vi "Add_to_speed_calib_file.vi"(2 "Desired Velocity":dbl format="%.2f", 3 "Max Velocity":dbl format="%.2f", 4 "New Row":dbl[](array[numeric]) format="%.2f", 5 "Max % Tweak allowable":dbl=40.0, 6 "Rig Name":string, 7 "Mode":enum16{"Add Row", "Get Error Value"}(ring)) -> (0 "Tweaked Demand":dbl format="%.4f", 1 "Calib Tweak %":dbl format="%.4f")   [LabVIEW 2022 SP3]
uses:
  Anemometry/Anemometry Sub Vis/File/Setup_Filetype.ctl
  Anemometry/Anemometry Sub Vis/Controls/In_Range.ctl
panel:
  out "XY Graph":T1(graph)
  out "Array":dbl[][](array[numeric]) format="%.4f"
  out "Channel Values":string[][](array[string])
  # "Dem Vel       Calib Tweak   Meas Vel"
  # "Dem V        Tweak      Weighting"
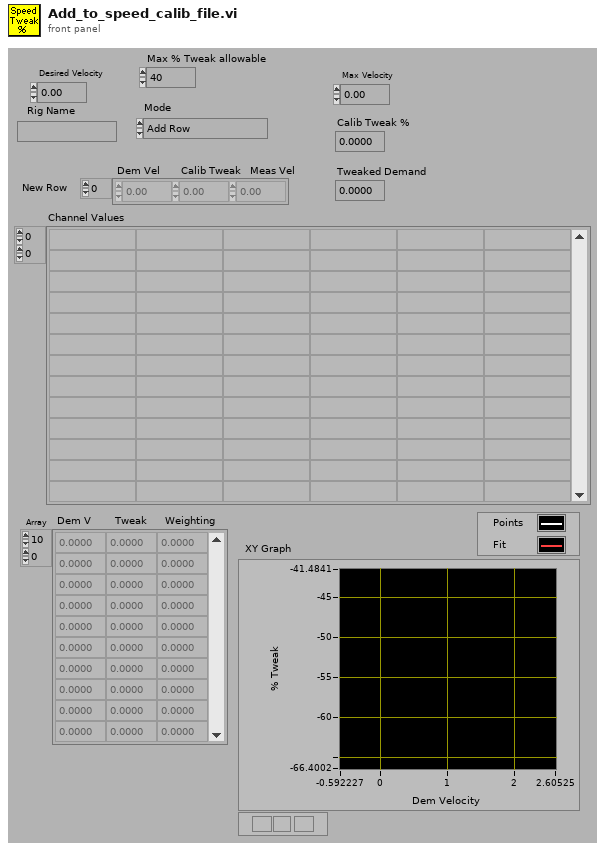
[diagram p1: front panel]
types:
  T1 = cluster{"t":dbl[], "Best Polynomial Fit":dbl[]}[]
  T2 = typedef "Setup_Filetype.ctl" = enum16{"Measurement Setups", "Calibration Setups", "General", "Results File Plotter Setups", "Speed Calib Tweaks"}
  T3 = typedef "In_Range.ctl" = enum16{"%", "±", "% & ±"}
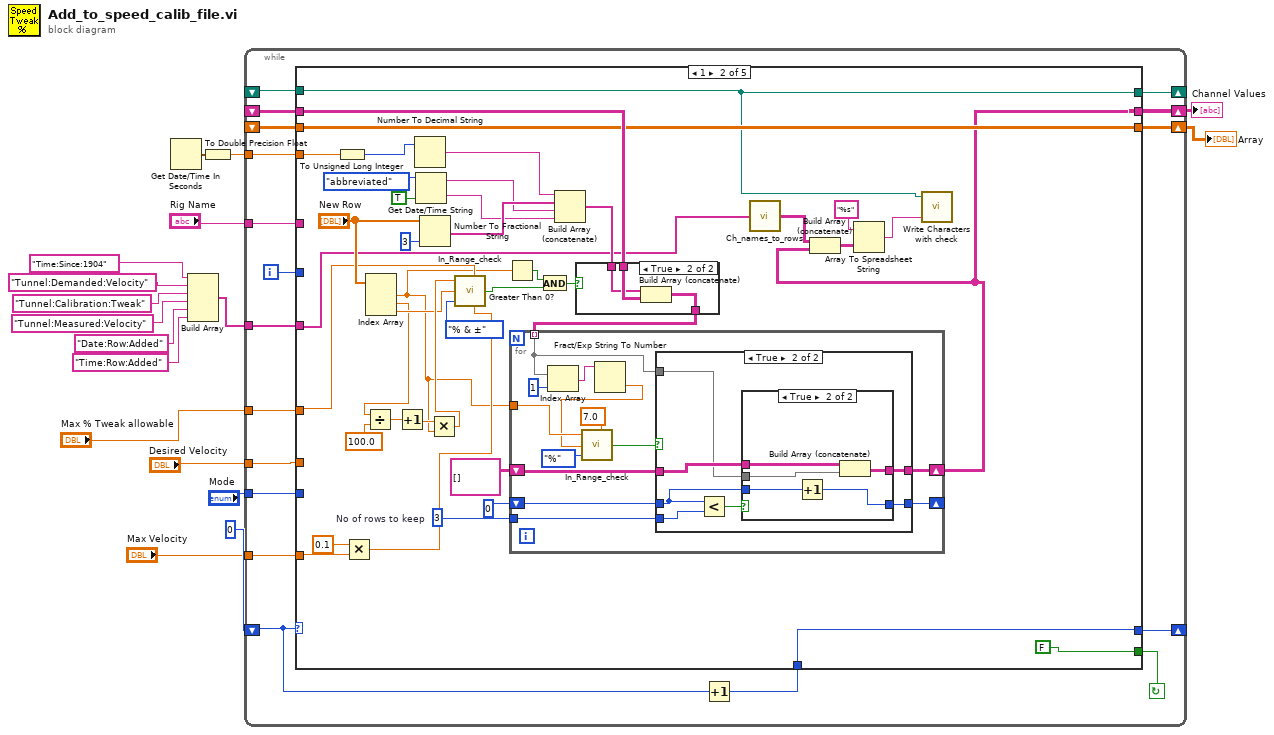
[diagram p0: block diagram]
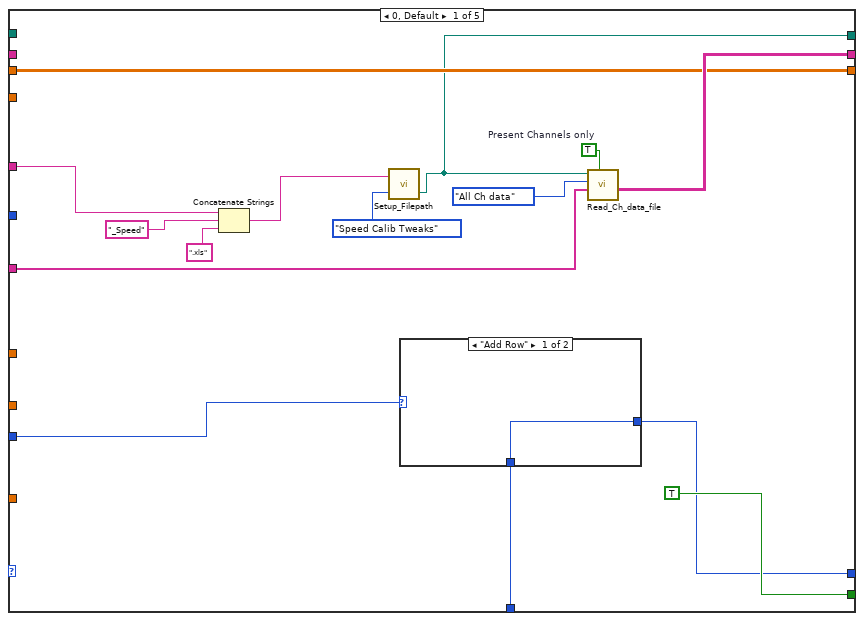
[diagram p2: hidden frame]
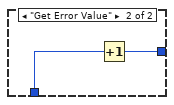
[diagram p3: hidden frame]
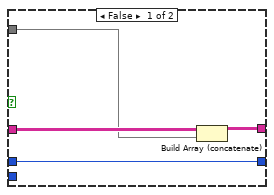
[diagram p5: hidden frame]
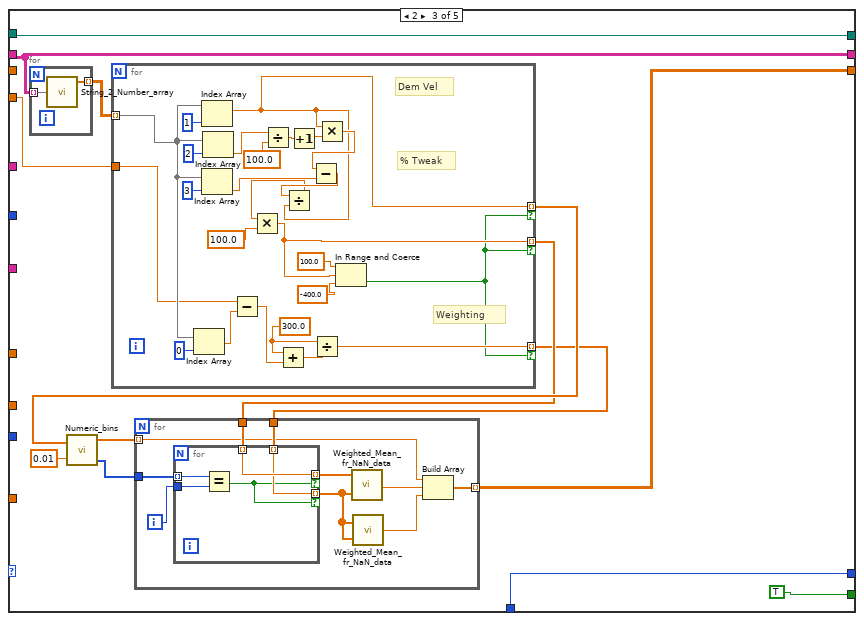
[diagram p7: hidden frame]
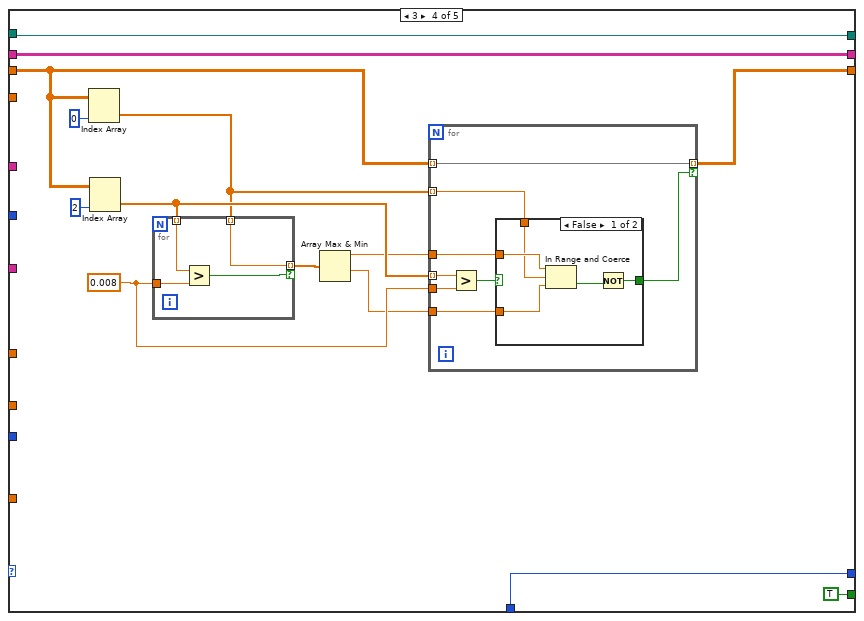
[diagram p8: hidden frame]
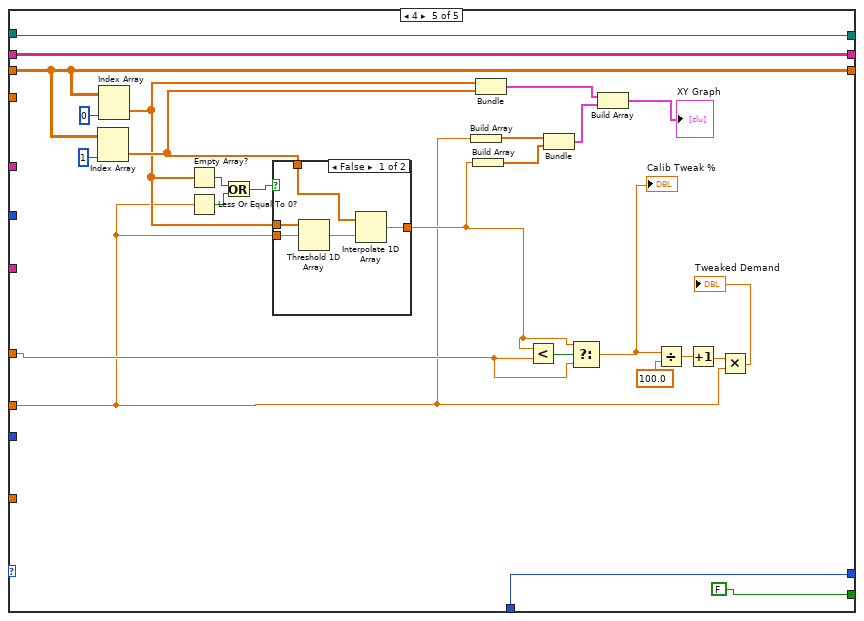
[diagram p10: hidden frame]
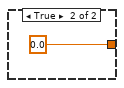
[diagram p11: hidden frame]
diagram:
  n1 = Get Date/Time In Seconds() -> (seconds since 1Jan1904=w4:timestamp)
  n2 = Build Array("Time:Since:1904" ("Substring"), "Tunnel:Demanded:Velocity" ("Substring"), "Tunnel:Calibration:Tweak" ("Substring"), "Tunnel:Measured:Velocity" ("Substring"), "Date:Row:Added" ("Substring"), "Time:Row:Added" ("Substring")) -> (w12:string[])
  n3 = To Double Precision Float(number=w4) -> (double precision float=w3:dbl)
  n4 = while {
    tunnel: "Max % Tweak allowable" -> [w20]
    tunnel: "Desired Velocity" -> [w21]
    tunnel: "Rig Name" -> [w22]
    shift-left: _ -> [w23]
    shift-right: [w24] -> w1
    tunnel: w12 -> [w30]
    shift-left: _ -> [w27]
    shift-right: [w28] -> w11
    shift-left: _ -> [w26]
    shift-right: [w29] -> _
    tunnel: "Mode" -> [w33]
    shift-left: 0 -> [w34]
    shift-right: [w32] -> _
    tunnel: "Max Velocity" -> [w19]
    tunnel: w3 -> [w18]
    i -> [w25]
    stop <- w35 continue-if-true
    n5 = Increment(x=w34) -> (x+1=w31:i32)
    n6 = case shown="1" w34 {
      tunnel: [TRUE FALSE TRUE TRUE FALSE] -> w35
      tunnel: w33 -> [w48 _ _ _ _]
      tunnel: [w47 w85 w138 w196 w239] -> w32
      tunnel: w31 -> [w46 w85 w138 w196 w239]
      tunnel: w30 -> [w45 w73 _ _ _]
      tunnel: [w36 w61 w141 w198 w242] -> w29
      tunnel: [w44 w72 w140 w197 w241] -> w28
      tunnel: w27 -> [_ w91 w140 w197 w241]
      tunnel: w26 -> [_ w61 w141 w198 w242]
      tunnel: w25 -> [_ _ _ _ _]
      tunnel: [w41 w89 w130 w185 w232] -> w24
      tunnel: w23 -> [w41 w89 _ w186 w232]
      tunnel: w22 -> [w40 _ _ _ _]
      tunnel: w21 -> [_ _ _ _ w217]
      tunnel: w20 -> [_ w68 _ _ w224]
      tunnel: w19 -> [_ w71 _ _ _]
      tunnel: w18 -> [_ w64 w139 _ _]
      frame 0, Default {
        w43 = TRUE  # Present Channels only
        n7 = Concatenate Strings(w40, "_Speed" ("Substring"), ".xls" ("string")) -> (w37:string)
        n8 = call "Setup_Filepath.vi"("Setup File Type"=Setup_Filetype."Speed Calib Tweaks", "Filename in"=w37) -> ("Filename Out"=w36:path)  [unwired: 1 out]
        n9 = case shown="\"Add Row\"" w48 {
          tunnel: [w51 w52] -> w47
          tunnel: w46 -> [w51 w53]
          frame "Add Row" {
          }
          frame "Get Error Value" {
            n10 = Increment(x=w53) -> (x+1=w52:i32)
          }
        }
        n11 = call "Read_Ch_data_file.vi"("Present Channels only"=w43, "Present Channels"=w45, "Output"=enum16{"All Ch data", "The last few rows"}."All Ch data", "Filename"=w36) -> ("Channel Values"=w44:string[][])  [unwired: 1 in, 4 out]
      }
      frame 1 {
        w83 = 3  # No of rows to keep
        n12 = To Unsigned Long Integer(number=w64) -> (unsigned 32bit integer=w82:u32)
        n13 = Multiply(x=0.1, y=w71) -> (x*y=w69:dbl)
        n14 = Index Array(array="New Row") -> (element #1=w58:dbl, element #2=w59:dbl, element #3=w62:dbl)  [unwired: 3 in]
        n15 = Divide(x=w59, y=100.0) -> (x/y=w66:dbl)
        n16 = Increment(x=w66) -> (x+1=w65:dbl)
        n17 = Number To Decimal String(number=w82) -> (decimal integer string=w92:string)  [unwired: 1 out]
        n18 = Get Date/Time String(date format (0)=enum16{"short", "long", "abbreviated"}."abbreviated", want seconds? (F)=TRUE) -> (date string=w80:string, time string=w79:string)  [unwired: 1 out]
        n19 = Number To Fractional String(number="New Row", precision (6)=i16 3) -> (F-format string=w88:string[])  [unwired: 2 out]
        n20 = Multiply(x=w65, y=w58) -> (x*y=w63:dbl)
        n21 = call "In_Range_check.vi"("±"=w69, "%"=w68, "Mode"=In_Range."% & ±", "Value"=w62, "Setpoint"=w63) -> ("In Range"=w57:bool)  [unwired: 2 out]
        n22 = Greater Than 0?(x=w58) -> (x > 0?=w56:bool)
        n23 = And(x=w56, y=w57) -> (x .and. y?=w55:bool)
        n24 = Build Array (concatenate)(w92, w88, w80, w79) -> (w90:string[])
        n25 = case shown="True" w55 {
          tunnel: w91 -> [w95 w98]
          tunnel: w90 -> [_ w97]
          tunnel: [w95 w96] -> w87
          frame False {
          }
          frame True {
            n26 = Build Array (concatenate)(w97, w98) -> (w96:string[][])
          }
        }
        n27 = for {
          tunnel: w58 -> [w110]
          tunnel: w87 -> [w104] mode=indexing
          shift-right: [w102] -> w72
          shift-left: string[][] [] -> [w103]
          shift-right: [w101] -> _
          shift-left: 0 -> [w100]
          tunnel: w83 -> [w99]
          n28 = Index Array(array=w104, index=1 ("Index")) -> (element=w108:string)
          n29 = Fract/Exp String To Number(string=w108) -> (number=w107:dbl)  [unwired: 4 out]
          n30 = call "In_Range_check.vi"("%"=7.0, "Mode"=In_Range."%", "Value"=w107, "Setpoint"=w110) -> ("In Range"=w105:bool)  [unwired: 1 in, 2 out]
          n31 = case shown="True" w105 {
            tunnel: w104 -> [w114 w120]
            tunnel: w103 -> [w115 w121]
            tunnel: [w113 w119] -> w102
            tunnel: [w112 w117] -> w101
            tunnel: w100 -> [w112 w118]
            tunnel: w99 -> [_ w116]
            frame False {
              n32 = Build Array (concatenate)(w115, w114) -> (w113:string[][])
            }
            frame True {
              n33 = Less?(x=w118, y=w116) -> (x < y?=w122:bool)
              n34 = case shown="True" w122 {
                tunnel: w121 -> [w124 w129]
                tunnel: w120 -> [_ w128]
                tunnel: [w124 w127] -> w119
                tunnel: w118 -> [w123 w126]
                tunnel: [w123 w125] -> w117
                frame False {
                }
                frame True {
                  n35 = Increment(x=w126) -> (x+1=w125:i32)
                  n36 = Build Array (concatenate)(w129, w128) -> (w127:string[][])
                }
              }
            }
          }
        }
        n37 = call "Ch_names_to_rows.vi"("Channel Names"=w73) -> ("3 Row names"=w76:string[][])
        n38 = Build Array (concatenate)(w76, w72) -> (w74:string[][])
        n39 = Array To Spreadsheet String(array=w74, 3:"%s" ("format string")) -> (spreadsheet string=w60:string)  [unwired: 1 out]
        n40 = call "Write Characters with check.vi"("String to Write"=w60, "file (use dialog)"=w61) -> ()  [unwired: 2 in, 1 out]
      }
      frame 2 {
        n41 = for {
          tunnel: w140 -> [w159] mode=indexing
          tunnel: [w158] -> w137 mode=indexing
          n42 = call "String_2_Number_array.vi"("Input String"=w159) -> ("Values"=w158:dbl[])
        }
        n43 = for {
          tunnel: w137 -> [w184] mode=indexing
          tunnel: w139 -> [w183]
          tunnel: [w162] -> w133 mode=indexing if=w160
          tunnel: [w163] -> w136 mode=indexing if=w160
          tunnel: [w161] -> w132 mode=indexing if=w160
          w167 = 300.0
          # "Weighting"
          # "% Tweak"
          # "Dem Vel"
          n44 = Index Array(array=w184, index=0 ("Index")) -> (element=w180:dbl)
          n45 = Index Array(array=w184, index=1 ("Index")) -> (element=w163:dbl)
          n46 = Index Array(array=w184, index=3 ("Index")) -> (element=w171:dbl)
          n47 = Index Array(array=w184, index=2 ("Index")) -> (element=w176:dbl)
          n48 = Subtract(x=w183, y=w180) -> (x-y=w166:dbl)
          n49 = Divide(x=w176, y=100.0) -> (x/y=w177:dbl)
          n50 = Add(x=w167, y=w166) -> (x+y=w168:dbl)
          n51 = Increment(x=w177) -> (x+1=w175:dbl)
          n52 = Divide(x=w167, y=w168) -> (x/y=w161:dbl)
          n53 = Multiply(x=w163, y=w175) -> (x*y=w172:dbl)
          n54 = Subtract(x=w172, y=w171) -> (x-y=w170:dbl)
          n55 = Divide(x=w170, y=w163) -> (x/y=w169:dbl)
          n56 = Multiply(x=w169, y=100.0) -> (x*y=w162:dbl)
          n57 = In Range and Coerce(upper limit=100.0, x=w162, lower limit=-400.0) -> (In Range?=w160:bool)  [unwired: 1 out]
        }
        n58 = call "Numeric_bins.vi"("Values"=w136, "Tolerance"=0.01) -> ("Bin Centres"=w131:dbl[], "Bin Index"=w134:i32[])  [unwired: 1 out]
        n59 = for {
          tunnel: w134 -> [w151]
          tunnel: w133 -> [w149]
          tunnel: w132 -> [w148]
          tunnel: w131 -> [w147] mode=indexing
          tunnel: [w145] -> w130 mode=indexing
          i -> [w152]
          n60 = for {
            tunnel: w152 -> [w157]
            tunnel: w151 -> [w156] mode=indexing
            tunnel: [w155] -> w150 mode=indexing if=w153
            tunnel: w149 -> [w155] mode=indexing
            tunnel: [w154] -> w144 mode=indexing if=w153
            tunnel: w148 -> [w154] mode=indexing
            n61 = Equal?(x=w156, y=w157) -> (x = y?=w153:bool)
          }
          n62 = call "Weighted_Mean_fr_NaN_data.vi"("Weighting"=w144, "Data"=w150) -> ("Mean value"=w146:dbl)
          n63 = call "Weighted_Mean_fr_NaN_data.vi"("Weighting"=w144, "Data"=w144) -> ("Mean value"=w143:dbl)
          n64 = Build Array(w147, w146, w143) -> (w145:dbl[])
        }
      }
      frame 3 {
        w191 = 0.008 ("y")
        n65 = Index Array(array=w186, index (col)=0 ("Index")) -> (element=w187:dbl[])  [unwired: 1 in]
        n66 = Index Array(array=w186, index (col)=2 ("Index")) -> (element=w190:dbl[])  [unwired: 1 in]
        n67 = for {
          tunnel: w190 -> [w216] mode=indexing
          tunnel: w187 -> [w215] mode=indexing
          tunnel: [w215] -> w192 mode=indexing if=w214
          tunnel: w191 -> [w213]
          n68 = Greater?(x=w216, y=w213) -> (0:w214:bool)
        }
        n69 = Array Max & Min(array=w192) -> (max value=w189:dbl, min value=w188:dbl)  [unwired: 2 out]
        n70 = for {
          tunnel: w191 -> [w206]
          tunnel: w190 -> [w205] mode=indexing
          tunnel: w189 -> [w203]
          tunnel: w188 -> [w202]
          tunnel: w187 -> [w201] mode=indexing
          tunnel: [w200] -> w185 mode=indexing if=w199
          tunnel: w186 -> [w200] mode=indexing
          n71 = Greater?(x=w205, y=w206) -> (0:w204:bool)
          n72 = case shown="False" w204 {
            selector: w204 -> [_ w212]
            tunnel: w203 -> [w211 _]
            tunnel: w202 -> [w210 _]
            tunnel: w201 -> [w209 _]
            tunnel: [w208 w212] -> w199
            frame False {
              n73 = In Range and Coerce(upper limit=w211, x=w209, lower limit=w210) -> (In Range?=w207:bool)  [unwired: 1 out]
              n74 = Not(x=w207) -> (.not. x?=w208:bool)
            }
            frame True {
            }
          }
        }
      }
      frame 4 {
        n75 = Index Array(array=w232, index (col)=1 ("Index")) -> (element=w226:dbl[])  [unwired: 1 in]
        n76 = Index Array(array=w232, index (col)=0 ("Index")) -> (element=w225:dbl[])  [unwired: 1 in]
        n77 = Empty Array?(array=w225) -> (empty?=w220:bool)
        n78 = Less Or Equal To 0?(x=w217) -> (x <= 0?=w219:bool)
        n79 = Or(x=w220, y=w219) -> (x .or. y?=w218:bool)
        n80 = case shown="False" w218 {
          tunnel: w217 -> [w247 _]
          tunnel: w226 -> [w245 _]
          tunnel: w225 -> [w244 _]
          tunnel: [w243 0.0] -> w221
          frame False {
            n81 = Threshold 1D Array(2:w247, 3:w244) -> (0:w246:dbl)  [unwired: 1 in]
            n82 = Interpolate 1D Array(1:w246, 2:w245) -> (0:w243:dbl)
          }
          frame True {
          }
        }
        n83 = Build Array(w217) -> (w223:dbl[])
        n84 = Build Array(w221) -> (w222:dbl[])
        n85 = Bundle(w225, w226) -> (w228:cluster{dbl[], dbl[]})  [unwired: 1 in]
        n86 = Less?(x=w221, y=w224) -> (x < y?=w231:bool)
        n87 = Bundle(w223, w222) -> (w229:cluster{dbl[], dbl[]})  [unwired: 1 in]
        n88 = Select(t=w221, s=w231, f=w224) -> (s? t:f=w230:dbl)
        "Calib Tweak %" <- w230
        n89 = Build Array(w228, w229) -> (→"XY Graph":cluster{dbl[], dbl[]}[])
        n90 = Divide(x=w230, y=100.0) -> (x/y=w235:dbl)
        n91 = Increment(x=w235) -> (x+1=w234:dbl)
        n92 = Multiply(x=w234, y=w217) -> (x*y=→"Tweaked Demand":dbl)
      }
    }
  }
  "Channel Values" <- w11
  "Array" <- w1
